vi "TCP Initialize Server - Local.vi"(8 "error in (no error)":errorcluster, 11 "Service Name":string) -> (0 "error out":errorcluster, 2 "TCP RX":refnum<user-event>, 3 "SLL Easy API via TCP out":refnum<class "SLL Easy API via TCP.lvclass">)   [LabVIEW 2016, in "SLL Easy API via TCP.lvclass"]
doc: "Initialize a TCP Server with the Provided Service Name"
uses:
  SLL Easy API via TCP.lvclass
  _Typedefs/TCP Event Data.ctl
  SLL Easy API via TCP.lvclass/SLL Easy API via TCP.ctl
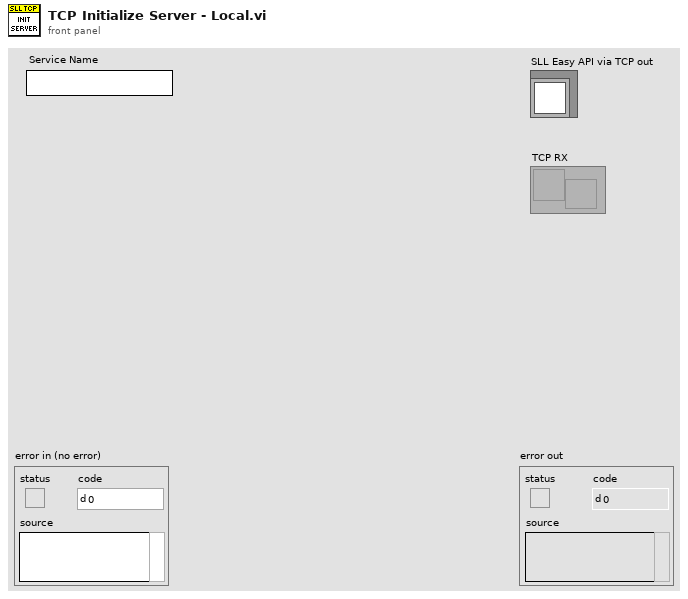
[diagram p1: front panel]
types:
  T1 = typedef "SLL Easy API via TCP.lvclass/User Events to TCP Engine.ctl" = cluster{"TCP RX":refnum<user-event>, "To TCP Engine":refnum<user-event>}
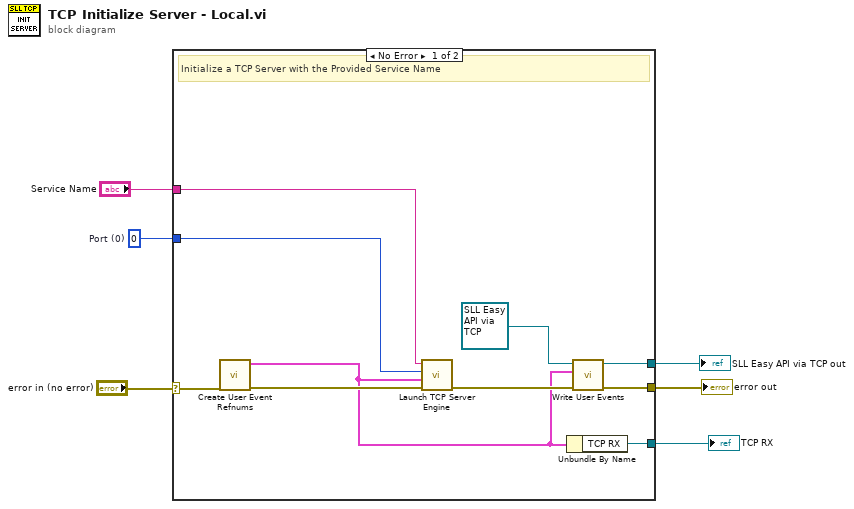
[diagram p0: block diagram]
diagram:
  w6 = 0  # Port (0)
  n1 = case shown="No Error" "error in (no error)" {
    selector: "error in (no error)" -> [w15 w17]
    tunnel: w6 -> [w8 _]
    tunnel: "Service Name" -> [w9 _]
    tunnel: [w16 _] -> w4
    tunnel: [w14 w17] -> w2
    tunnel: [w12 _] -> w1
    frame No Error {
      # "Initialize a TCP Server with the Provided Service Name"
      n2 = call "Create User Event Refnums.vi"("error in (no error)"=w15) -> ("error out"=w11:errorcluster, "User Events to TCP Engine"=w7:T1)  [unwired: 9 in]
      n3 = call "Launch TCP Server Engine.vi"("error in (no error)"=w11, "User Events"=w7, "Port (0)"=w8, "Service Name"=w9) -> ("error out"=w10:errorcluster)  [unwired: 7 in]
      n4 = Unbundle By Name(w7) -> ("TCP RX"=w16:refnum<user-event>)
      n5 = call "Write User Events.vi"("error in (no error)"=w10, "User Events to TCP Engine"=w7, "SLL Easy API via TCP in"=refnum<class "SLL Easy API via TCP.lvclass"> refnum ("SLL Easy API via TCP.lvclass")) -> ("error out"=w14:errorcluster, "SLL Easy API via TCP out"=w12:refnum<class "SLL Easy API via TCP.lvclass">)  [unwired: 7 in]
    }
    frame Error {
    }
  }
  "TCP RX" <- w4
  "error out" <- w2
  "SLL Easy API via TCP out" <- w1
